vi "update settings.vi"(8 "error in (no error)":errorcluster, 11 "Template in":refnum<class "Template.lvclass">) -> (0 "error out":errorcluster)   [LabVIEW 2020, in "Template.lvlib" / "Template.lvclass"]
doc: "This override is spun whenver the GUI controller requests the actor to show its settings user interface.\nWhen the configuration is changed, it generates a user event for the \"loop helper.vi\" that processes the new data defined by the user here and saves it as a JSON file"
uses:
  Template.lvclass
  Template.lvclass/Template.ctl
  read json file.vi
  build config path.vi
  read json file.vi/3c470e21-1639-4616-9875-34d8c0f16db8.vi
  read json file.vi/465192f6-cf10-4ed9-8c5f-bfc9042509a2.vi
  <vilib>/Utility/file.llb/Application Directory.vi
  tools/return class name.vi
  <userlib>/_OpenG.lib/file/file.llb/Create Dir if Non-Existant__ogtk.vi
  <vilib>/JDP Science/JSONtext/JSON text to Variant.vi
  <vilib>/JDP Science/JSONtext/Variant to JSON Text.vi
  <vilib>/Utility/error.llb/Error Cluster From Error Code.vi
  <vilib>/JDP Science/JSONtext/LVClass Serializer/JSONtext LVClass Serializer.lvclass
types:
  T1 = typedef "Template.lvlib/Template.lvclass/actor configuration.ctl" = cluster{"GlobalConfiguration":T2, "DeviceConfiguration":T3}
  T2 = typedef "Template.lvlib/Template.lvclass/shared actor configuration.ctl" = cluster{"DeviceFamily":string, "WriteData":bool, "BufferSize_samples":i32, "SyncDevice":bool, "ExecuteInterruptRoutine":bool, "InterruptRoutineTimeout_ms":i32}
  T3 = typedef "Template.lvlib/Template.lvclass/device configuration cluster.ctl" = cluster{"DeviceSpecificName":string, "HardwareReference":string, "UsedResources":T4[]}
  T4 = typedef "Template.lvlib/Template.lvclass/single resource cluster.ctl" = cluster{"ResourceLocation":string, "ResourceData":variant}
  T5 = typedef "Template.lvlib/Template.lvclass/base actor events.ctl" = cluster{"Stop Actor":refnum<user-event>, "New Error":refnum<user-event>, "New Settings":refnum<user-event>}
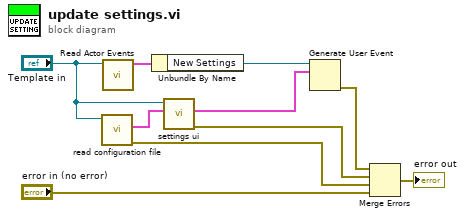
[diagram p0: block diagram]
diagram:
  n1 = call "read configuration file.vi"("Template in"="Template in") -> ("error out"=w1:errorcluster, "ActorConfiguration"=w4:T1)  [unwired: 9 in]
  n2 = call "Read Actor Events.vi"("Template in"="Template in") -> ("Base Actor Events"=w9:T5)  [unwired: 10 in]
  n3 = Unbundle By Name(w9) -> ("New Settings"=w8:refnum<user-event>)
  n4 = call-dynamic "settings ui.vi"("ActorConfiguration"=w4, "Template"="Template in") -> ("error out"=w5:errorcluster, "ActorConfiguration"=w3:T1)  [unwired: 8 in]
  n5 = Generate User Event(user event=w8, event data cluster=w3) -> (error out=w6:errorcluster)  [unwired: 2 in, 1 out]
  n6 = Merge Errors(w6, w5, w1, "error in (no error)") -> (→"error out":errorcluster)
